vi "PLL_PID.vi"() -> ()   [LabVIEW 2018]
doc: "Please ensure that at least one period is generated or else the measurement VIs do not work properly."
uses:
  <vilib>/measure/matone.llb/Extract Single Tone Information 1 Chan.vi
  <vilib>/addons/control/pid/pid.llb/PID (DBL).vi
  <vilib>/measure/NI_MABase.lvlib
  <vilib>/Analysis/NI_AALPro.lvlib
  <vilib>/measure/NI_MAPro.lvlib
  <vilib>/addons/control/pid/NI_PID_pid.lvlib
panel:
  in  "signal type":T1(ring)
  in  "output range":cluster{"output high":dbl, "output low":dbl}={"output high"=100.0, "output low"=-100.0} {"output low" format="%.2f"; "output high" format="%.2f"}
  out "Numeric":dbl
  in  "PID_Phase":T2={"proportional gain (Kc)"=0.1, "integral time (Ti, min)"=0.0008, "derivative time (Td, min)"=0.0} {"derivative time (Td, min)" format="%.3f"; "integral time (Ti, min)" items=["Take a Coffee"=0.1, "Yawning"=0.01, "Take a Deep Breath"=0.001, "Normal"=0.0008, "A Little Bit Fast"=0.0001, "Fast"=1e-05, "Too Fast"=1e-06]; "proportional gain (Kc)" format="%.3f"}
  out "Current Frequency [Hz]":dbl=10.000000000000004 format="%.2f"
  in  "PID_Frequency":T2={"proportional gain (Kc)"=0.9, "integral time (Ti, min)"=0.0008, "derivative time (Td, min)"=0.0} {"derivative time (Td, min)" format="%.3f"; "integral time (Ti, min)" items=["Take a Coffee"=0.1, "Yawning"=0.01, "Take a Deep Breath"=0.001, "Normal"=0.0008, "A Little Bit Fast"=0.0001, "Fast"=1e-05, "Too Fast"=1e-06]; "proportional gain (Kc)" format="%.3f"}
  out "Waveform Graph":waveform(dbl)[](graph)=[{"t0"=timestamp(0 s since 1904-01-01), "dt"=0.001, "Y"=array[1000 elements]}, {"t0"=timestamp(0 s since 1904-01-01), "dt"=0.001, "Y"=array[1000 elements]}]
  in  "stop":bool
  in  "sampling info":cluster{"Fs":dbl, "#s":dbl}={"Fs"=1000.0, "#s"=1000.0} {"Fs" format="%.2p"}
  in  "Desired Frequency [Hz]":dbl=10.0 format="%_6f"
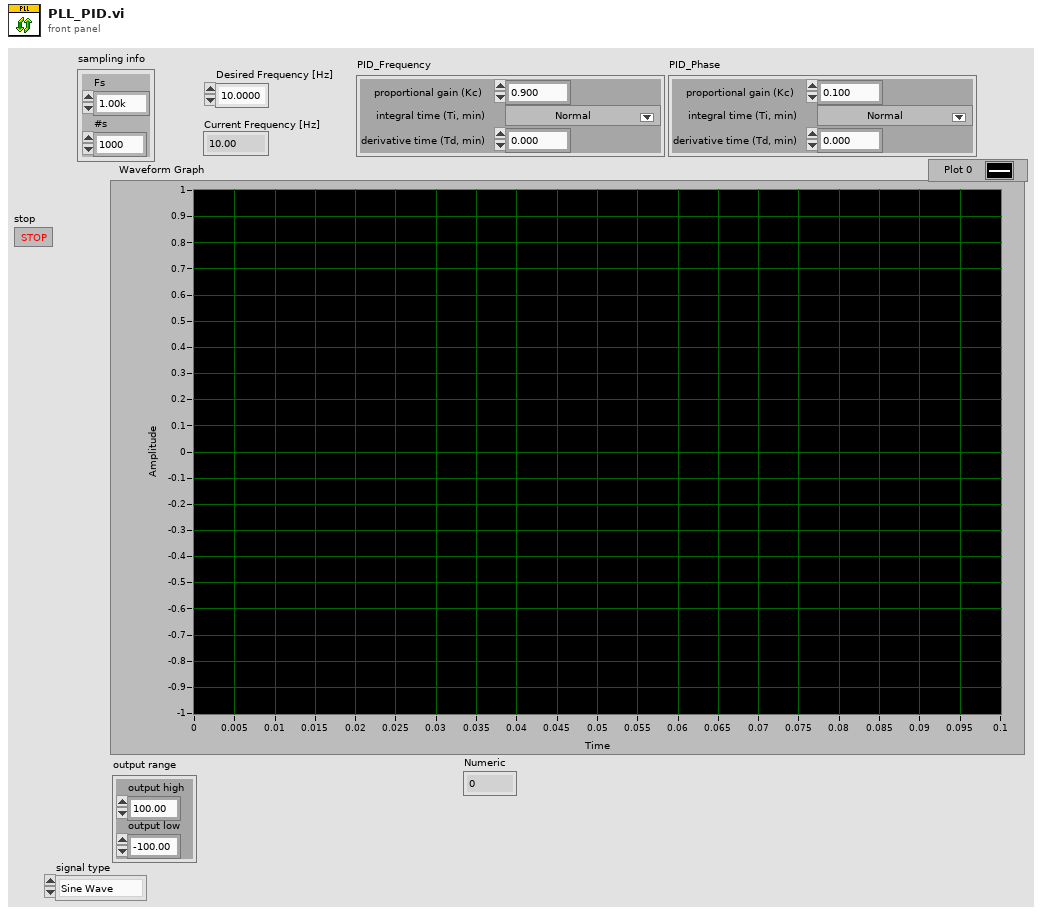
[diagram p1: front panel]
types:
  T1 = enum16{"Sine Wave", "Triangle Wave", "Square Wave", "Sawtooth Wave"}
  T2 = cluster{"proportional gain (Kc)":dbl, "integral time (Ti, min)":dbl, "derivative time (Td, min)":dbl}
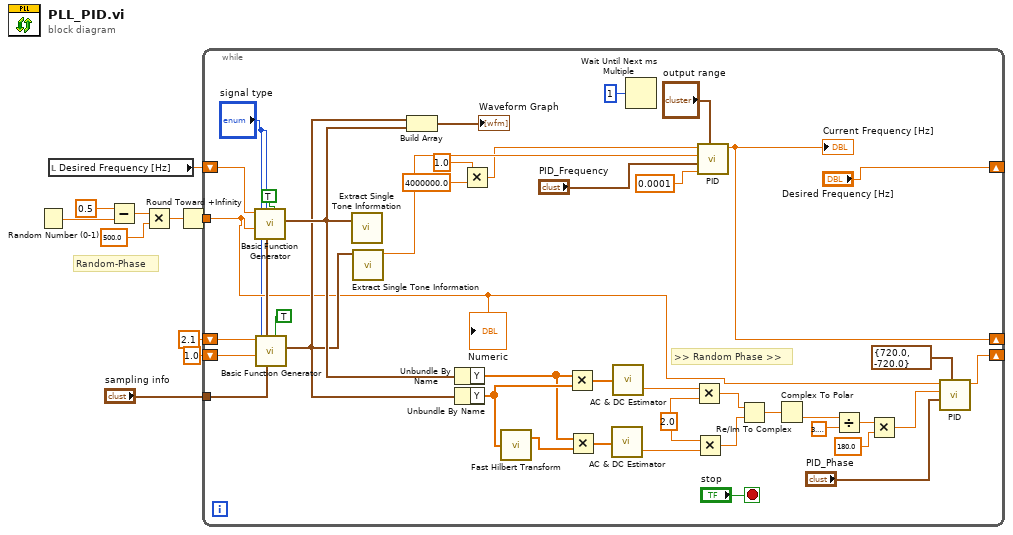
[diagram p0: block diagram]
diagram:
  # "Random-Phase"
  n1 = Random Number (0-1)() -> (number: 0 to 1=w8:dbl)
  n2 = local read "Desired Frequency [Hz]"() -> (w1:dbl)
  n3 = Subtract(x=0.5, y=w8) -> (x-y=w2:dbl)
  n4 = Multiply(x=w2, y=500.0) -> (x*y=w5:dbl)
  n5 = Round Toward +Infinity(x=w5) -> (ceil(x): smallest int >= x=w4:dbl)
  n6 = while {
    tunnel: "sampling info" -> [w51]
    shift-right: [w19] -> _
    shift-left: 1.0 -> [w32]
    tunnel: w4 -> [w15]
    shift-right: [w22] -> _
    shift-left: 2.1 ("f") -> [w46]
    shift-right: ["Desired Frequency [Hz]"] -> _
    shift-left: w1 -> [w25]
    stop <- "stop" stop-if-true
    w30 = 2.0 ("x")
    # ">> Random Phase >>"
    n7 = call <vilib>:"Basic Function Generator.vi"("reset signal"=TRUE, "sampling info"=w51, "signal type"="signal type", "phase"=w15, "frequency"=w25) -> ("signal out"=w29:waveform(dbl))  [unwired: 4 in, 2 out]
    n8 = call <vilib>:"Basic Function Generator.vi"("reset signal"=TRUE, "sampling info"=w51, "signal type"="signal type", "phase"=w32, "frequency"=w46) -> ("signal out"=w28:waveform(dbl))  [unwired: 4 in, 2 out]
    n9 = call-poly <vilib>:"Extract Single Tone Information.vi"("time signal in"=w29) -> ()  [unwired: 5 in, 6 out]
    n10 = call-poly <vilib>:"Extract Single Tone Information.vi"("time signal in"=w28) -> ("detected frequency"=w24:dbl)  [unwired: 5 in, 5 out]
    n11 = Build Array(w28, w29) -> (→"Waveform Graph":waveform(dbl)[])
    n12 = Unbundle By Name(w29) -> ("Y"=w43:dbl[])
    n13 = Unbundle By Name(w28) -> ("Y"=w45:dbl[])
    n14 = Multiply(x=1.0, y=4000000.0) -> (x*y=w16:dbl)
    n15 = call <vilib>:"Fast Hilbert Transform.vi"("X"=w45) -> ("Hilbert{X}"=w44:dbl[])  [unwired: 1 out]
    n16 = Multiply(x=w43, y=w45) -> (x*y=w42:dbl[])
    n17 = Multiply(x=w43, y=w44) -> (x*y=w41:dbl[])
    n18 = call <vilib>:"AC & DC Estimator.vi"("Signal (V)"=w41) -> ("DC estimate (V)"=w40:dbl)  [unwired: 1 out]
    n19 = call <vilib>:"AC & DC Estimator.vi"("Signal (V)"=w42) -> ("DC estimate (V)"=w31:dbl)  [unwired: 1 out]
    n20 = Wait Until Next ms Multiple(millisecond multiple=u32 1) -> ()  [unwired: 1 out]
    n21 = Multiply(x=w31, y=w30) -> (x*y=w34:dbl)
    n22 = Multiply(x=w30, y=w40) -> (x*y=w33:dbl)
    n23 = call-poly <vilib>:"PID.vi"("output range"="output range", "dt (s)"=0.0001, "PID gains"="PID_Frequency", "process variable"=w24, "setpoint"=w16) -> ("output"=w22:dbl)  [unwired: 5 in, 1 out]
    "Current Frequency [Hz]" <- w22
    n24 = Re/Im To Complex(1:w33, 2:w34) -> (0:w35:cdb)
    n25 = Complex To Polar(r * e^(i*theta)=w35) -> (theta=w36:dbl)  [unwired: 1 out]
    n26 = Divide(x=w36, y=3.141592653589793) -> (x/y=w38:dbl)
    n27 = Multiply(x=w38, y=180.0) -> (x*y=w20:dbl)
    n28 = call-poly <vilib>:"PID.vi"("output range"=cluster{"output high":dbl, "output low":dbl} {"output high"=720.0, "output low"=-720.0}, "PID gains"="PID_Phase", "process variable"=w20, "setpoint"=w15) -> ("output"=w19:dbl)  [unwired: 6 in, 1 out]
    "Numeric" <- w15
  }
